vi "AmpControl.vi"() -> ()   [LabVIEW 2009]
uses:
  <vilib>/DAQmx/write.llb/DAQmx Write (Analog DBL 1Chan 1Samp).vi
  <vilib>/DAQmx/write.llb/DAQmx Write (Digital Bool 1Line 1Point).vi
panel:
  in  "Gain":dbl(slide) scale=0.0..10.0
  in  "Gate":bool
  in  "stop":bool
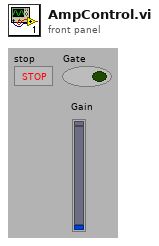
[diagram p1: front panel]
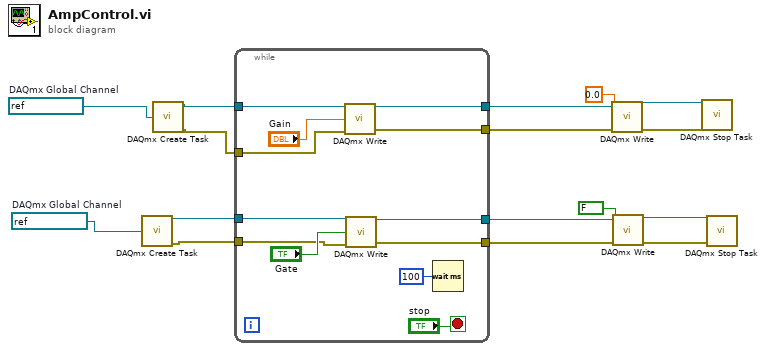
[diagram p0: block diagram]
diagram:
  w6 = refnum<k21> "AOD Gate"  # DAQmx Global Channel
  w3 = refnum<k21> "AOD Gain"  # DAQmx Global Channel
  n1 = call <vilib>:"DAQmx Create Task.vi"("global virtual channels"=w6) -> ("task out"=w5:refnum<k21>, "error out"=w4:errorcluster)  [unwired: 4 in, 9 out]
  n2 = call <vilib>:"DAQmx Create Task.vi"("global virtual channels"=w3) -> ("task out"=w2:refnum<k21>, "error out"=w1:errorcluster)  [unwired: 4 in, 9 out]
  n3 = while {
    tunnel: w5 -> [w26]
    tunnel: w2 -> [w25]
    tunnel: w1 -> [w22]
    tunnel: w4 -> [w21]
    tunnel: [w20] -> w16
    tunnel: [w19] -> w14
    tunnel: [w18] -> w13
    tunnel: [w17] -> w12
    stop <- "stop" stop-if-true
    n4 = call-poly <vilib>:"DAQmx Write.vi"("task/channels in"=w25, "data"="Gain", "error in"=w22) -> ("task out"=w20:refnum<k21>, "error out"=w19:errorcluster)  [unwired: 1 in, 10 out]
    n5 = call-poly <vilib>:"DAQmx Write.vi"("task/channels in"=w26, "data"="Gate", "error in"=w21) -> ("task out"=w18:refnum<k21>, "error out"=w17:errorcluster)  [unwired: 1 in, 10 out]
    n6 = Wait (ms)(milliseconds to wait=u32 100) -> ()  [unwired: 1 out]
  }
  n7 = call-poly <vilib>:"DAQmx Write.vi"("task/channels in"=w16, "data"=0.0, "error in"=w14) -> ("task out"=w10:refnum<k21>, "error out"=w9:errorcluster)  [unwired: 1 in, 10 out]
  n8 = call-poly <vilib>:"DAQmx Write.vi"("task/channels in"=w13, "data"=FALSE, "error in"=w12) -> ("task out"=w8:refnum<k21>, "error out"=w7:errorcluster)  [unwired: 1 in, 10 out]
  n9 = call <vilib>:"DAQmx Stop Task.vi"("task/channels in"=w10, "error in"=w9) -> ()  [unwired: 14 out]
  n10 = call <vilib>:"DAQmx Stop Task.vi"("task/channels in"=w8, "error in"=w7) -> ()  [unwired: 14 out]
